vi "Read Output.vi"(8 "error in (no error)":errorcluster, 11 "UIStep in":refnum<class "UIStep.lvclass">) -> (0 "error out":errorcluster, 2 "Output":T1[](array[typedef]), 3 "UIStep out":refnum<class "UIStep.lvclass">)   [LabVIEW 2015, in "UIStep.lvclass"]
uses:
  UIStep.lvclass
  Step/STEP_OUTPUT.ctl
  Step/OUTPUT_DATA_TYPE.ctl
  OutputUI/OUTPUT_CHECK_TYPE.ctl
  Step/OUTPUT_VALUE_TYPE.ctl
  Step.lvclass
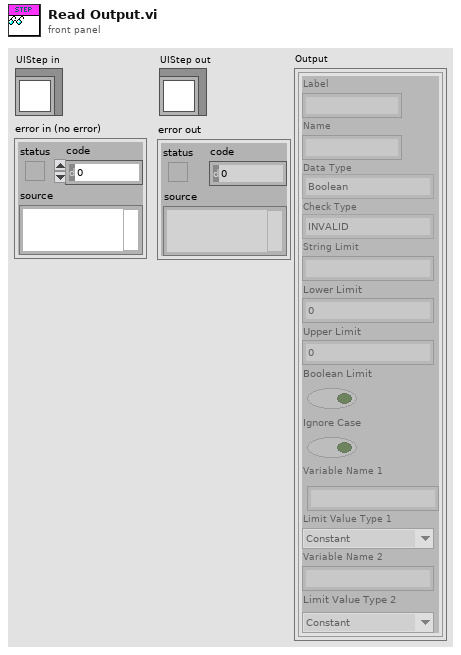
[diagram p1: front panel]
types:
  T1 = typedef "Step.lvclass/STEP_OUTPUT.ctl" = cluster{"Label":string, "Name":string, "Data Type":T2, "Check Type":T3, "String Limit":string, "Lower Limit":dbl, "Upper Limit":dbl, "Boolean Limit":bool, "Ignore Case":bool, "Variable Name 1":string, "Limit Value Type 1":T4, "Variable Name 2":string, "Limit Value Type 2":T4}
  T2 = typedef "Step.lvclass/OUTPUT_DATA_TYPE.ctl" = enum16{"Boolean", "String", "Numeric", "Other"}
  T3 = typedef "Step.lvclass/OUTPUT_CHECK_TYPE.ctl" = enum16{"INVALID", "DO_NOT_CHECK", "RECORD", "VARIABLE", "EQUAL", "NOT_EQUAL", "STR_CONTAINS", "STR_START_WITH", "STR_END_WITH", "STR_REGEX_MATCH", "NUM_GT", "NUM_LT", "NUM_GE", "NUM_LE", "NUM_RANGE", "NUM_RANGE_BDY"}
  T4 = typedef "Step.lvclass/OUTPUT_VALUE_TYPE.ctl" = enum16{"Constant", "Variable"}
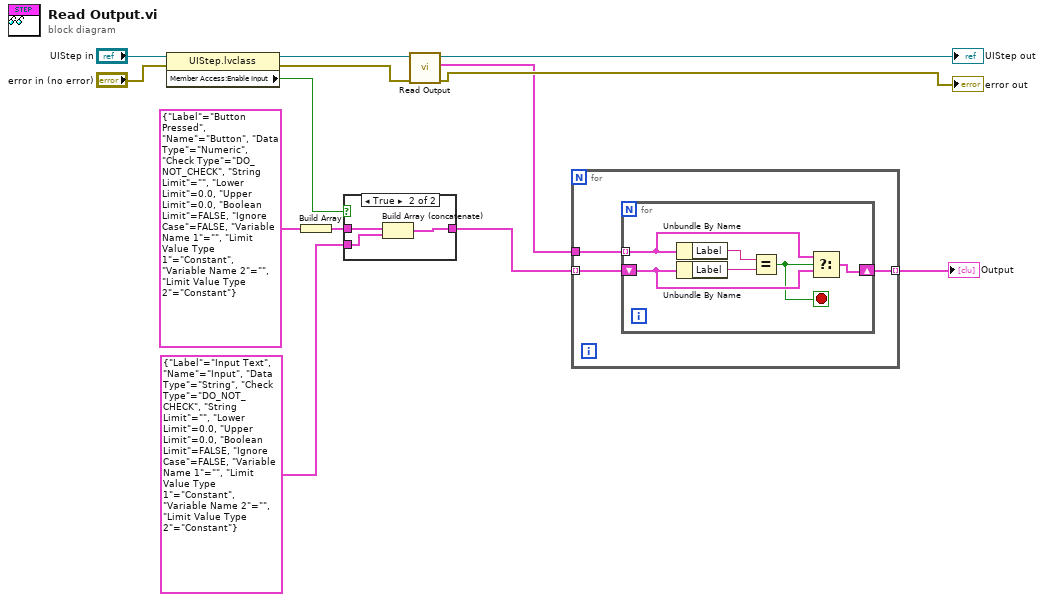
[diagram p0: block diagram]
diagram:
  n1 = property class="UIStep.lvclass"(reference="UIStep in", error in="error in (no error)") -> (reference out=w7:refnum<class "UIStep.lvclass">, error out=w6:errorcluster, "Member Access:Enable Input"=w4:bool)
  n2 = Build Array(T1 {"Label"="Button Pressed", "Name"="Button", "Data Type"=enum."Numeric", "Check Type"=enum."DO_NOT_CHECK", "String Limit"="", "Lower Limit"=0.0, "Upper Limit"=0.0, "Boolean Limit"=FALSE, "Ignore Case"=FALSE, "Variable Name 1"="", "Limit Value Type 1"=enum."Constant", "Variable Name 2"="", "Limit Value Type 2"=enum."Constant"} ("Output")) -> (w3:T1[])
  n3 = case shown="True" w4 {
    tunnel: w3 -> [w14 w17]
    tunnel: T1 {"Label"="Input Text", "Name"="Input", "Data Type"=enum."String", "Check Type"=enum."DO_NOT_CHECK", "String Limit"="", "Lower Limit"=0.0, "Upper Limit"=0.0, "Boolean Limit"=FALSE, "Ignore Case"=FALSE, "Variable Name 1"="", "Limit Value Type 1"=enum."Constant", "Variable Name 2"="", "Limit Value Type 2"=enum."Constant"} ("Output") -> [_ w16]
    tunnel: [w14 w15] -> w1
    frame False {
    }
    frame True {
      n4 = Build Array (concatenate)(w17, w16) -> (w15:T1[])
    }
  }
  n5 = call-parent "Read Output.vi"("error in (no error)"=w6, "Step in"=w7) -> ("error out"=→"error out":errorcluster, "Output"=w10:T1[], "Step out"=→"UIStep out":refnum<class "UIStep.lvclass">)  [unwired: 7 in]
  n6 = for {
    tunnel: w1 -> [w19] mode=indexing
    tunnel: w10 -> [w20]
    tunnel: [w18] -> w11 mode=indexing
    n7 = for {
      tunnel: w20 -> [w24] mode=indexing
      shift-right: [w22] -> w18
      shift-left: w19 -> [w23]
      stop <- w21 stop-if-true
      n8 = Unbundle By Name(w24) -> ("Label"=w25:string)
      n9 = Unbundle By Name(w23) -> ("Label"=w26:string)
      n10 = Equal?(x=w25, y=w26) -> (x = y?=w21:bool)
      n11 = Select(t=w24, s=w21, f=w23) -> (s? t:f=w22:T1)
    }
  }
  "Output" <- w11
